vi "NI VeriStand - Open Single Waveform Read Session (DBL).vi"(7 "Communication Properties":T2, 8 "error in (no error)":errorcluster, 11 "DBL Waveform Data Reference":T1) -> (0 "error out":errorcluster, 3 "Single Waveform Read Session (DBL)":refnum<class "Single Waveform Read (DBL).lvclass">)   [LabVIEW 2020, in "NI_VS Custom Device Waveform API.lvlib" / "Single Waveform Read (DBL).lvclass"]
doc: "Opens a session for reading data from or writing data to a specific waveform or waveforms associated with a custom device. You must manually select the instance to use according to the number of waveforms with which you want to interact, whether the data type of the waveforms is DBL or CDB, and whether you want to read or write waveform data."
uses:
  Single Waveform Read (DBL).lvclass
  D:/p4/penguin/lvaddon/Veristand/master/src/LabVIEW/vilib/NI VeriStand/Custom Device Waveform API/Waveform Session.lvclass
  Communication Properties.ctl
  Custom Device API/Waveform Data Reference.ctl
  Access mode.ctl
  Internal Comm Classes/WPL Comm/WPL Comm (1D DBL)/WPL Comm (1D DBL).lvclass
  Single Waveform Read (DBL).lvclass/Single Waveform Read (DBL).ctl
  Waveform Session.lvclass/Waveform Session.ctl
  Waveform Session.lvclass
  NI_VS Custom Device Waveform API.lvlib
  Custom Device API/Custom Device API.lvlib
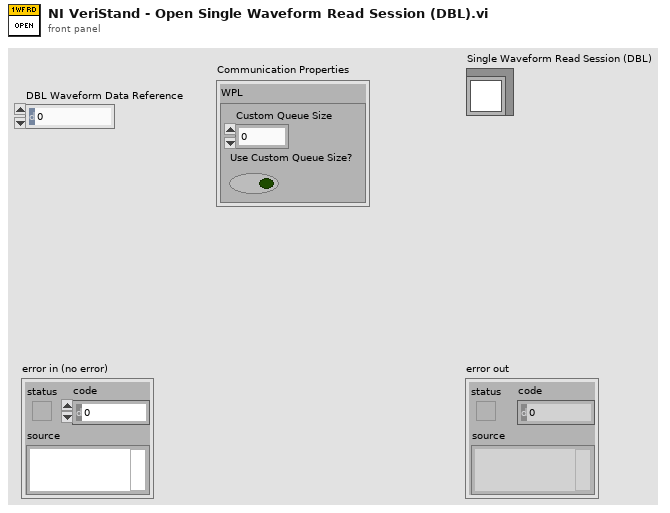
[diagram p1: front panel]
types:
  T1 = typedef "Custom Device API.lvlib/Waveform Data Reference.ctl" = i32
  T2 = typedef "NI_VS Custom Device Waveform API.lvlib/Communication Properties.ctl" = cluster{"WPL":cluster{"Custom Queue Size":i32, "Use Custom Queue Size?":bool}}
  T3 = typedef "NI_VS Custom Device Waveform API.lvlib/Access mode.ctl" = enum16{"Read", "Write"}
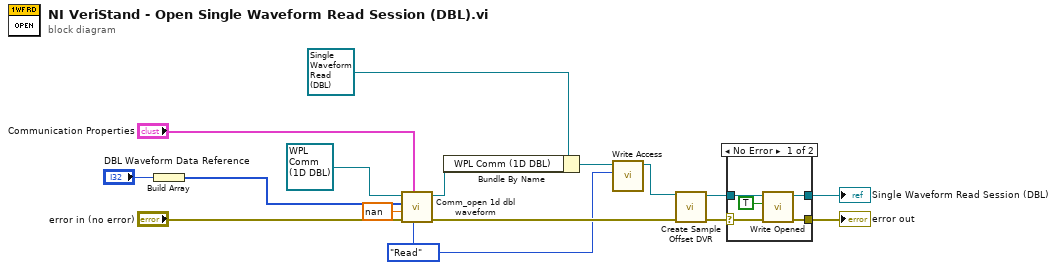
[diagram p0: block diagram]
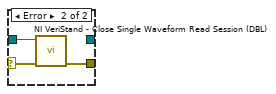
[diagram p2: hidden frame]
diagram:
  w1 = Access_mode."Read" ("Access")
  n1 = Build Array("DBL Waveform Data Reference") -> (w5:T1[])
  n2 = call "Comm_open 1d dbl waveform.vi"("Access"=w1, "Communication Properties"="Communication Properties", "error in (no error)"="error in (no error)", "dt"=nan, "WFM Data Ref"=w5, "WPL Comm (1D DBL) in"=refnum<class "WPL Comm (1D DBL).lvclass"> refnum ("Internal Comm Classes.lvlib:WPL Comm (1D DBL).lvclass")) -> ("error out"=w14:errorcluster, "WPL Comm (1D DBL) out"=w9:refnum<class "WPL Comm (1D DBL).lvclass">)  [unwired: 4 in]
  n3 = Bundle By Name(cluster=refnum<class "Single Waveform Read (DBL).lvclass"> refnum, "WPL Comm (1D DBL)"=w9) -> (w3:refnum<class "Single Waveform Read (DBL).lvclass">)
  n4 = call "Write Access.vi"("Access"=w1, "Waveform Session in"=w3) -> ("Waveform Session out"=w2:refnum<class "Single Waveform Read (DBL).lvclass">)  [unwired: 9 in]
  n5 = call "Create Sample Offset DVR.vi"("error in (no error)"=w14, "Waveform Session in"=w2) -> ("error out"=w12:errorcluster, "Waveform Session out"=w13:refnum<class "Single Waveform Read (DBL).lvclass">)  [unwired: 8 in]
  n6 = case shown="No Error" w12 {
    selector: w12 -> [w20 w23]
    tunnel: [w20 w22] -> w16
    tunnel: w13 -> [w19 w21]
    tunnel: [w18 _] -> w15
    frame No Error {
      n7 = call "Write Opened.vi"("Opened"=TRUE, "Waveform Session in"=w19) -> ("Waveform Session out"=w18:refnum<class "Single Waveform Read (DBL).lvclass">)  [unwired: 9 in]
    }
    frame Error {
      n8 = call "NI VeriStand - Close Single Waveform Read Session (DBL).vi"("error in (no error)"=w23, "Single Waveform Read Session (DBL)"=w21) -> ("error out"=w22:errorcluster)  [unwired: 9 in]
    }
  }
  "error out" <- w16
  "Single Waveform Read Session (DBL)" <- w15
